vi "fetch buffer.vi"(8 "error in":errorcluster, 11 "sample queue":T1) -> (0 "error out":errorcluster, 1 "empty?":bool, 2 "Time Stamp":timestamp, 3 "data table":T2)   [LabVIEW 2013, in "TDMS datalogger runtime.lvclass"]
uses:
  TDMS datalogger runtime.lvclass
  <vilib>/NI/Tag Bus/table/data table.ctl
  sample queue.ctl
  <vilib>/NI/Tag Bus/table/data table.lvlib
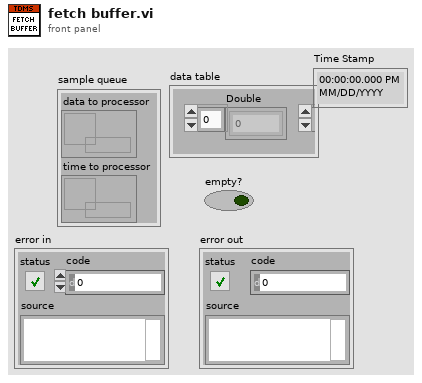
[diagram p1: front panel]
types:
  T1 = typedef "TDMS datalogger runtime.lvclass/sample queue.ctl" = cluster{"data to processor":refnum<queue>, "time to processor":refnum<queue>}
  T2 = typedef "tag bus.lvlib/data table.lvlib/data table.ctl" = cluster{"Double":dbl[], "Single":sgl[], "I64":i64[], "I32":i32[], "I16":i16[], "I8":i8[], "U64":u64[], "U32":u32[], "U16":u16[], "U8":u8[], "Boolean":bool[], "String":string[], "Array of Double":cluster{"DBL Array":dbl[]}[], "Array of Single":cluster{"SGL Array":sgl[]}[], "Array of I64":cluster{"I64 Array":i64[]}[], "Array of I32":cluster{"I32 Array":i32[]}[], "Array of I16":cluster{"I16 Array":i16[]}[], "Array of I8":cluster{"I8 Array":i8[]}[], "Array of U64":cluster{"U64 Array":u64[]}[], "Array of U32":cluster{"U32 Array":u32[]}[], "Array of U16":cluster{"U16 Array":u16[]}[], "Array of U8":cluster{"U8 Array":u8[]}[], "Array of Boolean":cluster{"Boolean Array":bool[]}[], "Array of String":cluster{"String Array":string[]}[]}
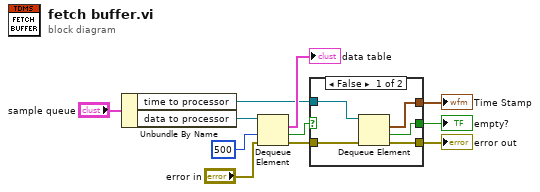
[diagram p0: block diagram]
diagram:
  n1 = Unbundle By Name("sample queue") -> ("time to processor"=w2:refnum<queue>, "data to processor"=w7:refnum<queue>)
  n2 = Dequeue Element(queue=w7, timeout in ms (-1)=500, error in (no error)="error in") -> (element=→"data table":T2, timed out?=w6:bool, error out=w3:errorcluster)  [unwired: 1 out]
  n3 = case shown="False" w6 {
    selector: w6 -> [_ w18]
    tunnel: [w16 w18] -> w5
    tunnel: [w14 w17] -> w4
    tunnel: w3 -> [w15 w17]
    tunnel: w2 -> [w13 _]
    tunnel: [w12 _] -> w1
    frame False {
      n4 = Dequeue Element(queue=w13, error in (no error)=w15) -> (element=w12:timestamp, timed out?=w16:bool, error out=w14:errorcluster)  [unwired: 1 in, 1 out]
    }
    frame True {
    }
  }
  "error out" <- w4
  "empty?" <- w5
  "Time Stamp" <- w1
